vi "Motor_InitParam.vi"(0 "Motor Control In":refnum<class "MotorControl.lvclass">, 1 "Force Rate Limit (N/min)":cluster{"ForceRateLow":dbl, "ForceRateHigh":dbl}={"ForceRateLow"=600.0, "ForceRateHigh"=10000.0} {"ForceRateHigh" format="%#_13g"; "ForceRateLow" format="%#_13g"}, 2 "Motor Quantity":i32=8, 3 "PID gain schedule":T1(array[cluster]), 5 "MotorConstant(F/V)":dbl, 7 "PID Loop Period":dbl=-1.0 format="%#_13g", 9 "FrictionModel":cluster{"Coeff+":dbl[], "Coeff-":dbl[]}, 11 "error in (no error)":errorcluster, 12 "output range (N)":cluster{"output high":dbl, "output low":dbl}={"output high"=100.0, "output low"=0.0}, 13 "TransferRatio":dbl=1.0 format="%#_13g", 14 "setpoint range (A)":cluster{"setpoint high":dbl, "setpoint low":dbl}={"setpoint high"=0.75, "setpoint low"=-0.2}) -> (4 "Motor Control Out":refnum<class "MotorControl.lvclass">, 15 "error out":errorcluster)   [LabVIEW 2015, in "MotorControl.lvclass"]
uses:
  MotorControl.lvclass
  MotorControl.lvclass/MotorControl.ctl
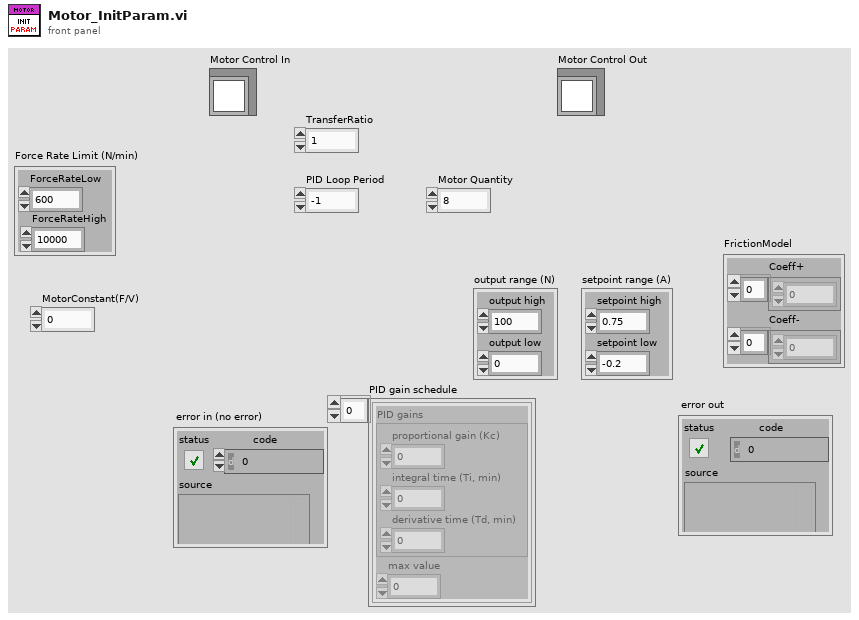
[diagram p1: front panel]
types:
  T1 = cluster{"PID gains":cluster{"proportional gain (Kc)":dbl, "integral time (Ti, min)":dbl, "derivative time (Td, min)":dbl}, "max value":dbl}[]
  T2 = cluster{"setpoint high":dbl, "setpoint low":dbl}[]
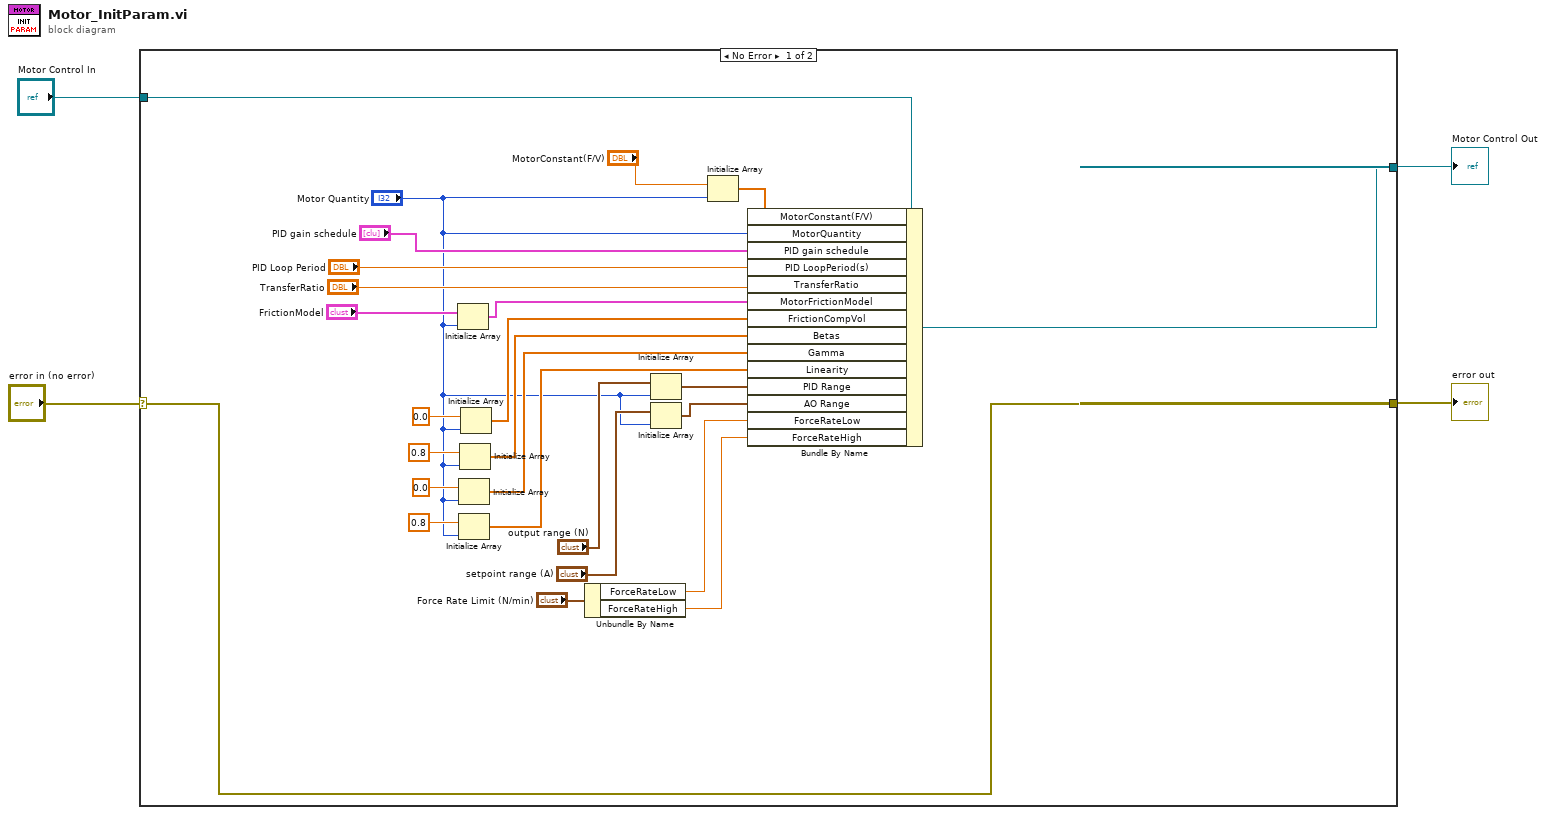
[diagram p0: block diagram]
diagram:
  n1 = case shown="No Error" "error in (no error)" {
    selector: "error in (no error)" -> [w25 w32]
    tunnel: [w25 w32] -> w3
    tunnel: "Motor Control In" -> [w26 w31]
    tunnel: [w27 w31] -> w1
    frame No Error {
      n2 = Initialize Array("FrictionModel", "Motor Quantity") -> (w10:cluster{"Coeff+":dbl[], "Coeff-":dbl[]}[])
      n3 = Initialize Array(0.0 ("element"), "Motor Quantity") -> (w14:dbl[])
      n4 = Initialize Array(0.8 ("element"), "Motor Quantity") -> (w11:dbl[])
      n5 = Initialize Array(0.8 ("element"), "Motor Quantity") -> (w22:dbl[])
      n6 = Initialize Array(0.0 ("element"), "Motor Quantity") -> (w30:dbl[])
      n7 = Unbundle By Name("Force Rate Limit (N/min)") -> ("ForceRateLow"=w16:dbl, "ForceRateHigh"=w15:dbl)
      n8 = Initialize Array("output range (N)", "Motor Quantity") -> (w24:cluster{"output high":dbl, "output low":dbl}[])
      n9 = Initialize Array("setpoint range (A)", "Motor Quantity") -> (w23:T2)
      n10 = Initialize Array("MotorConstant(F/V)", "Motor Quantity") -> (w5:dbl[])
      n11 = Bundle By Name(cluster=w26, "MotorConstant(F/V)"=w5, "MotorQuantity"="Motor Quantity", "PID gain schedule"="PID gain schedule", "PID LoopPeriod(s)"="PID Loop Period", "TransferRatio"="TransferRatio", "MotorFrictionModel"=w10, "FrictionCompVol"=w30, "Betas"=w22, "Gamma"=w14, "Linearity"=w11, "PID Range"=w24, "AO Range"=w23, "ForceRateLow"=w16, "ForceRateHigh"=w15) -> (w27:refnum<class "MotorControl.lvclass">)
    }
    frame Error {
    }
  }
  "error out" <- w3
  "Motor Control Out" <- w1
